vi "Set_Field.vi"() -> ()   [LabVIEW 2013]
uses:
  <instrlib>/Mercury iXX/Public/Controls/Comms Transport Layer.ctl
  <instrlib>/Mercury iXX/Public/Controls/Serial Settings.ctl
  <instrlib>/Mercury iXX/Public/Controls/ISOBus Address.ctl
  <instrlib>/Mercury iXX/Public/Libraries/Magnet/Controls/Identifier.ctl
  <instrlib>/Mercury iXX/Public/Controls/Unit String.ctl
  <instrlib>/Mercury iXX/Public/Controls/Is Valid LED.ctl
  <instrlib>/Mercury iXX/Public/Libraries/System/Open/Open System.vi
  <instrlib>/Mercury iXX/Public/Libraries/System/Read/Catalogue (Read).vi
  <instrlib>/Mercury iXX/Public/Libraries/Magnet/Open/Open Magnet Device.vi
  <instrlib>/Mercury iXX/Public/Libraries/Magnet/Signals/Read/Field (Read).vi
  <instrlib>/Mercury iXX/Public/Libraries/Magnet/Signals/Set/Target Field (Set).vi
  <instrlib>/Mercury iXX/Mercury iXX.lvlib
  <instrlib>/Mercury iXX/Public/Libraries/System.lvlib
  <instrlib>/Mercury iXX/Public/Libraries/Magnet.lvlib
panel:
  out "Response":string
  out "Valid?":T1
  in  "Set Unit":T2="T"
  in  "Set Field (T)":dbl format="%.4g"
  in  "stop":bool
  out "error out":errorcluster
  out "Unit":T2
  out "Field":dbl
  in  "Device Identifier":T3="GRPZ"
  in  "ISOBUS address":T4=-1 caption="ISOBUS address (-1)"
  out "Devices":string[](array[string])
  in  "Clear Previous Connections (False)":bool
  in  "ID Query (True)":bool
  in  "Serial Configuration":T5={"Baud Rate"=9600, "Parity"=0, "Data Bits"=8, "Stop Bits"=10, "Flow Control"=0} {"Flow Control" items=["None", "XON/XOFF", "RTS/CTS", "XON/XOFF & RTS/CTS", "DTR/DSR", "XON/XOFF & DTR/DSR"]; "Stop Bits" items=["1.0"=10, "2.0"=20]; "Data Bits" items=["7"=7, "8"=8]; "Parity" items=["None", "Odd", "Even"]; "Baud Rate" items=["300"=300, "600"=600, "1200"=1200, "2400"=2400, "4800"=4800, "9600"=9600, "19200"=19200]}
  in  "Comms Layer":T6
  in  "IP Address":string
  in  "VISA resource name":refnum<visa-resource-name>
  # "Field Read"
  # "Field Set"
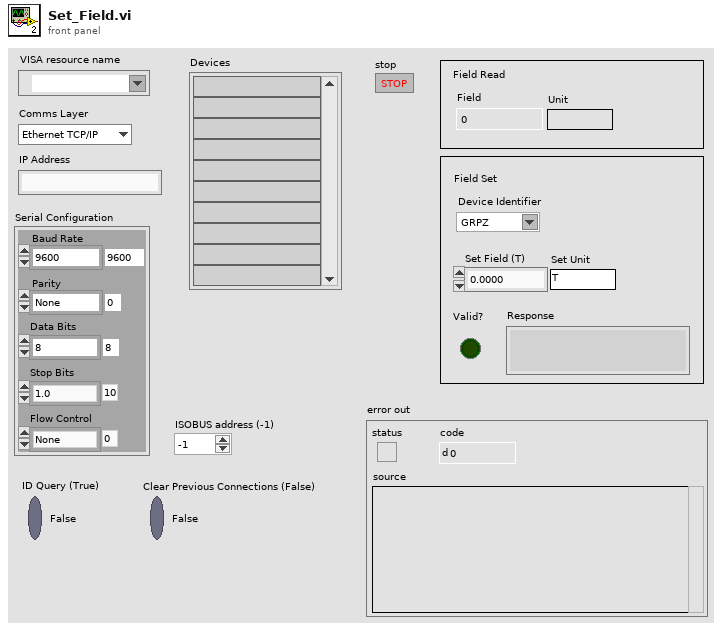
[diagram p1: front panel]
types:
  T1 = typedef "Mercury iXX.lvlib/Is Valid LED.ctl" = bool
  T2 = typedef "Mercury iXX.lvlib/Unit String.ctl" = string
  T3 = typedef "Mercury iXX.lvlib/Magnet.lvlib/Identifier.ctl" = string
  T4 = typedef "Mercury iXX.lvlib/ISOBus Address.ctl" = i32
  T5 = typedef "Mercury iXX.lvlib/Serial Settings.ctl" = cluster{"Baud Rate":u32, "Parity":u16, "Data Bits":u16, "Stop Bits":u16, "Flow Control":u16}
  T6 = typedef "Mercury iXX.lvlib/Comms Transport Layer.ctl" = enum16{"Ethernet TCP/IP", "USB", "ISOBus - RS-232", "GPIB"}
  T7 = typedef "Mercury iXX.lvlib/Mercury Reference.ctl" = cluster{"Comms":refnum<visa-resource-name>, "Device ID":string[], "Comms Layer":T6, "Command":string, "Query reference":T8}
  T8 = typedef "Mercury iXX.lvlib/Query Dynamic Reference.ctl" = refnum<vi>
  T9 = typedef "Mercury iXX.lvlib/Response String.ctl" = string
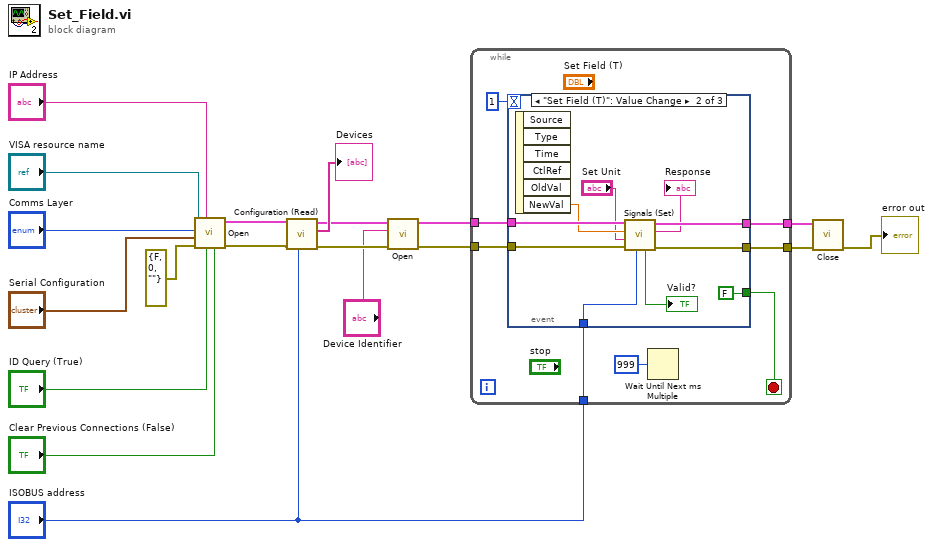
[diagram p0: block diagram]
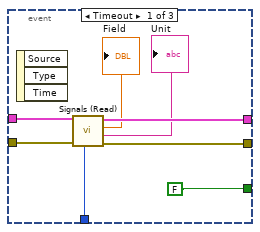
[diagram p2: hidden frame]
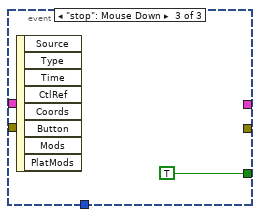
[diagram p3: hidden frame]
diagram:
  n1 = call-poly <instrlib>:"Open.vi"("Clear Previous Connections (False)"="Clear Previous Connections (False)", "ID Query (True)"="ID Query (True)", "IP Address"="IP Address", "error in (no error)"=errorcluster {"status"=FALSE, "code"=0, "source"=""}, "Serial Configuration"="Serial Configuration", "Comms Layer"="Comms Layer", "VISA resource name"="VISA resource name") -> ("error out"=w11:errorcluster, "Mercury Reference Out"=w12:T7)  [unwired: 3 out]
  n2 = call-poly <instrlib>:"Configuration (Read).vi"("ISOBUS address"="ISOBUS address", "error in"=w11, "Mercury Reference In"=w12) -> ("error out"=w8:errorcluster, "Devices"=→"Devices":string[], "Mercury Reference Out"=w9:T7)  [unwired: 5 in, 1 out]
  n3 = call-poly <instrlib>:"Open.vi"("error in (no error)"=w8, "Device Identifier"="Device Identifier", "Mercury Reference In"=w9) -> ("error out"=w5:errorcluster, "Mercury Reference Out"=w6:T7)  [unwired: 7 in]
  n4 = while {
    tunnel: w6 -> [w27]
    tunnel: w5 -> [w26]
    tunnel: "ISOBUS address" -> [w25]
    tunnel: [w24] -> w3
    tunnel: [w23] -> w2
    stop <- w20 stop-if-true
    n5 = event shown="[1] \"Set Field (T)\": Value Change" {
      selector: _ -> [_ _ _]
      dyn-events: _ -> [_ _ _]
      timeout: 1 -> [_ _ _]
      tunnel: w27 -> [w35 w45 _]
      tunnel: w26 -> [w34 w42 _]
      tunnel: w25 -> [w33 w40 _]
      tunnel: [w32 w43 _] -> w24
      tunnel: [w31 w41 _] -> w23
      tunnel: [FALSE FALSE TRUE] -> w20
      event Timeout {
        n6 = event-data() -> ()  [unwired: 1 in, 3 out]
        n7 = call-poly <instrlib>:"Signals (Read).vi"("ISOBUS address"=w33, "error in"=w34, "Mercury Reference In"=w35) -> ("error out"=w31:errorcluster, "Unit"=→"Unit":T2, "Field"=→"Field":dbl, "Mercury Reference Out"=w32:T7)  [unwired: 4 in, 1 out]
      }
      event "Set Field (T)": Value Change {
        n8 = event-data() -> ("NewVal"=w44:dbl)  [unwired: 1 in, 5 out]
        n9 = call-poly <instrlib>:"Signals (Set).vi"("ISOBUS address"=w40, "error in"=w42, "Unit"="Set Unit", "Target Field"=w44, "Mercury Reference In"=w45) -> ("error out"=w41:errorcluster, "Response"=→"Response":T9, "Mercury Reference Out"=w43:T7, "Valid?"=→"Valid?":T1)  [unwired: 3 in]
      }
      event "stop": Mouse Down {
        n10 = event-data() -> ()  [unwired: 1 in, 8 out]
      }
    }
    n11 = Wait Until Next ms Multiple(millisecond multiple=u32 999) -> ()  [unwired: 1 out]
  }
  n12 = call <instrlib>:"Close.vi"("error in (no error)"=w2, "Mercury Reference"=w3) -> ("error out"=→"error out":errorcluster)  [unwired: 9 in]
